vi "checksum(SubVI).vi"(11 "String":string) -> (3 "Numeric":u8)   [LabVIEW 2012]
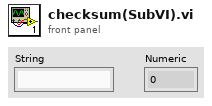
[diagram p1: front panel]
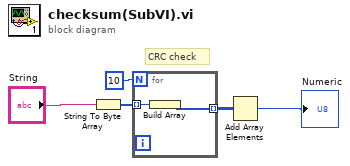
[diagram p0: block diagram]
diagram:
  # "CRC check"
  n1 = String To Byte Array(string="String") -> (unsigned byte array=w1:u8[])
  n2 = for {
    N: 10 -> [_]
    tunnel: w1 -> [w7] mode=indexing
    tunnel: [w6] -> w3 mode=indexing
    n3 = Build Array(w7) -> (w6:u8[])
  }
  n4 = Add Array Elements(numeric array=w3) -> (sum=→"Numeric":u8)
